vi "ini_file.vi"(0 "device_type in":refnum<class "device_type.lvclass">, 11 "error in (no error)":errorcluster) -> (4 "device_type out":refnum<class "device_type.lvclass">, 6 "number of pulses":i32, 15 "error out":errorcluster)   [LabVIEW 2021, in "device_type.lvclass"]
uses:
  device_type.lvclass
  device_type.lvclass/device_type.ctl
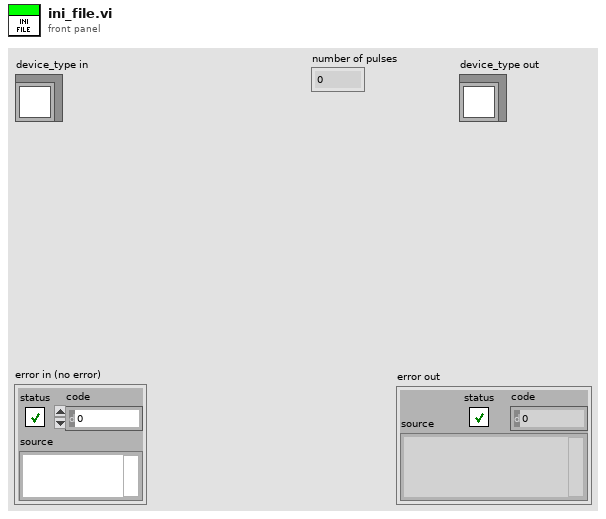
[diagram p1: front panel]
types:
  T1 = enum16{"open", "open or create", "create or replace", "create", "open (read-only)"}
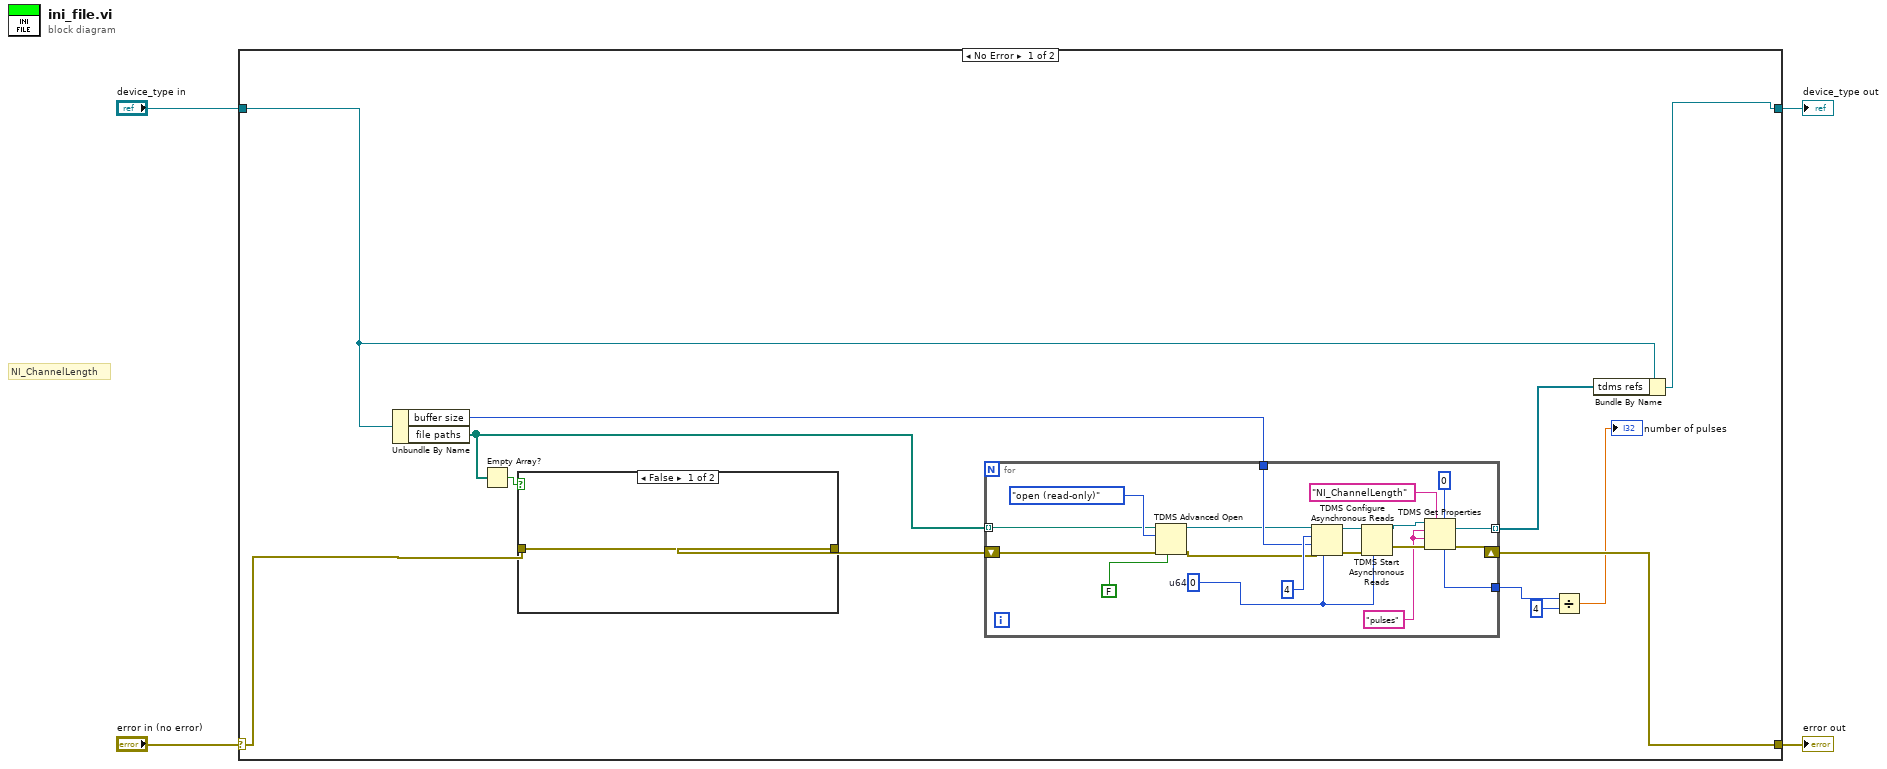
[diagram p0: block diagram]
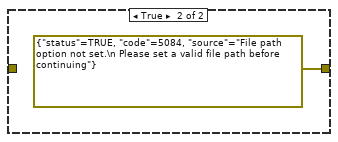
[diagram p2: hidden frame]
diagram:
  # "NI_ChannelLength"
  n1 = case shown="No Error" "error in (no error)" {
    selector: "error in (no error)" -> [w8 w39]
    tunnel: [w9 w39] -> w3
    tunnel: [w10 w38] -> w1
    tunnel: "device_type in" -> [w11 w38]
    frame No Error {
      n2 = Unbundle By Name(w11) -> ("buffer size"=w16:u32, "file paths"=w13:path[])
      n3 = Empty Array?(array=w13) -> (empty?=w14:bool)
      n4 = case shown="False" w14 {
        tunnel: [w17 errorcluster {"status"=TRUE, "code"=5084, "source"="File path option not set.\n Please set a valid file path before continuing"} ("error in (no error)")] -> w12
        tunnel: w8 -> [w17 _]
        frame False {
        }
        frame True {
        }
      }
      n5 = for {
        tunnel: w13 -> [w27] mode=indexing
        tunnel: [w23] -> w15 mode=indexing
        shift-right: [w24] -> w9
        shift-left: w12 -> [w32]
        tunnel: w16 -> [w30]
        tunnel: [w20] -> w7
        w19 = "pulses" ("channel name")
        w31 = u64 0  # u64
        n6 = TDMS Advanced Open(6:FALSE ("Disable Buffering? (T)"), 8:w32, 10:T1."open (read-only)" ("Operation"), 11:w27) -> (0:w33:errorcluster, 3:w29:refnum<k34>)  [unwired: 1 in, 1 out]
        n7 = TDMS Configure Asynchronous Reads(6:w31, 8:w33, 9:w30, 10:u32 4 ("Number of Buffers (4)"), 11:w29) -> (0:w35:errorcluster, 3:w28:refnum<k34>)  [unwired: 1 in]
        n8 = TDMS Start Asynchronous Reads(6:w31, 8:w35, 11:w28) -> (0:w25:errorcluster, 3:w26:refnum<k34>)  [unwired: 1 in]
        n9 = TDMS Get Properties(5:u64 0, 7:"NI_ChannelLength" ("property name"), 8:w25, 9:w19, 10:w19, 11:w26) -> (0:w24:errorcluster, 3:w23:refnum<k34>, 4:w20:u64)  [unwired: 3 out]
      }
      n10 = Divide(x=w7, y=u64 4) -> (x/y=→"number of pulses":dbl)
      n11 = Bundle By Name(cluster=w11, "tdms refs"=w15) -> (w10:refnum<class "device_type.lvclass">)
    }
    frame Error {
    }
  }
  "error out" <- w3
  "device_type out" <- w1
